vi "Main_N5224Bv5_beta.vi"() -> ()   [LabVIEW 2020]
uses:
  <instrlib>/Agilent PNA Series/Agilent PNA Series.lvlib
  Chamber_2018/ControlCluster.ctl
panel:
  out "Numeric 2":dbl
  out "Numeric":dbl
  in  "Tab Control":enum32{"Setup", "Results"}(tab)
  in  "File Path:":path=path "C:/Users/LAB543-Chamber/Desktop/meas/TEST.txt"
  in  "Saved by":string
  in  "File Description:":string
  out "error":errorcluster={"status"=FALSE, "code"=1073676294, "source"="VISA Read in MotorBack 2(SubVI).vi->Main_E8361C_2.vi"}
  in  "Cluster":T1={"Power Level"=-5.0, "Center Freq"=28000000000.0, "Span Freq"=2000000000.0, "Sweep Points"=5, "IF Bandwidth"=500.0, "Average Count"=5, "error"={"status"=FALSE, "code"=0, "source"=""}, "Instrument"="USB0::0x2A8D::0x2A01::MY58422353::INSTR", "Mode"=0, "Motor Range"=360, "Motor Step"=10, "VISA"="COM4"} {"Motor Step" items=["0.5 deg"=1, "1 deg"=2, "3 deg"=6, "5 deg"=10, "10 deg"=20]; "Motor Range" items=["360 deg"=360, "180 deg"=180]; "Mode" items=["Create", "Delete", "Select"]; "IF Bandwidth" format="%.3p"; "Span Freq" format="%.3p"; "Center Freq" format="%.3p"; "Power Level" format="%.2p"}
  out "Progress Bar":dbl(slide)=0.0055248618784530384 scale=0.0..1.0
  out "Gain array":dbl[][](array[numeric]) format="%#.3p"
  out "Gain Patten":dbl[][](graph)
  out "Phase array":dbl[][](array[numeric]) format="%#.3p"
  out "CurrentGain":dbl[](array[numeric])
  out "CurrentPhase":dbl[](array[numeric])
  # "Hz"
  # "Hz"
  # "Hz"
  # "dBm"
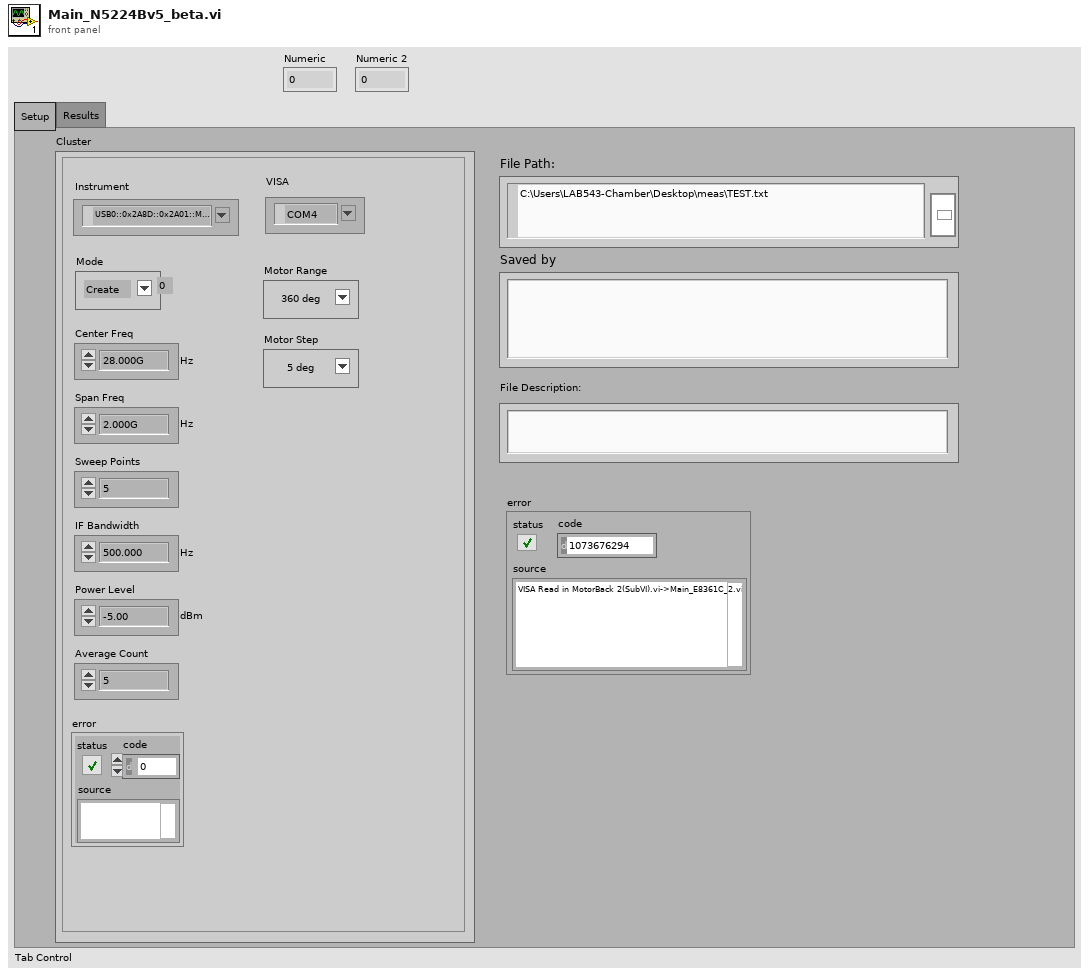
[diagram p1: front panel]
types:
  T1 = typedef "ControlCluster.ctl" = cluster{"Power Level":dbl, "Center Freq":dbl, "Span Freq":dbl, "Sweep Points":u32, "IF Bandwidth":dbl, "Average Count":i32, "error":errorcluster, "Instrument":refnum<visa-resource-name>, "Mode":u16, "Motor Range":u16, "Motor Step":u16, "VISA":refnum<visa-resource-name>}
  T2 = typedef "visaerror.ctl" = errorcluster
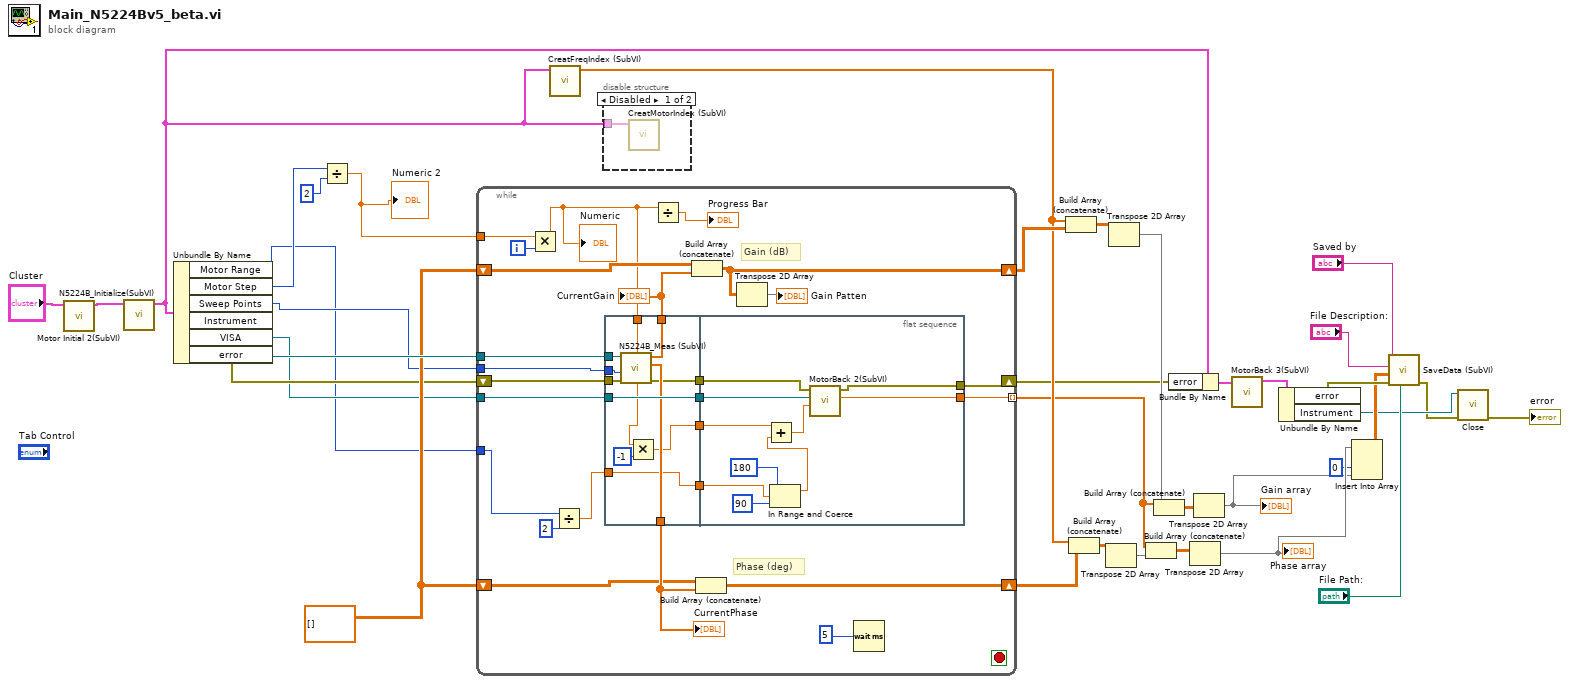
[diagram p0: block diagram]
diagram:
  w35 = dbl[][] []
  n1 = call "Motor Initial 2(SubVI).vi"("Cluster in 2"="Cluster") -> ("Cluster in 3"=w9:T1)  [unwired: 10 in]
  n2 = call "N5224B_Initialize(SubVI).vi"("Cluster in"=w9) -> ("Cluster out"=w16:T1)  [unwired: 10 in]
  n3 = Unbundle By Name(w16) -> ("Motor Range"=w2:u16, "Motor Step"=w8:u16, "Sweep Points"=w10:u32, "Instrument"=w36:refnum<visa-resource-name>, "VISA"=w6:refnum<visa-resource-name>, "error"=w7:errorcluster)
  n4 = Divide(x=w8, y=u16 2) -> (x/y=w3:dbl)
  "Numeric 2" <- w3
  n5 = while {
    tunnel: w36 -> [w61]
    shift-right: [w53] -> w33
    shift-left: w35 -> [w59]
    shift-right: [w57] -> w31
    shift-left: w35 -> [w56]
    shift-right: [w45] -> w5
    shift-left: w7 -> [w60]
    tunnel: w6 -> [w51]
    tunnel: w10 -> [w46]
    tunnel: w3 -> [w43]
    tunnel: w2 -> [w38]
    tunnel: [w37] -> w1 mode=indexing
    i -> [w49]
    stop <- _ stop-if-true
    # "Gain (dB)"
    # "Phase (deg)"
    n6 = Multiply(x=w43, y=w49) -> (x*y=w42:dbl)
    "Numeric" <- w42
    n7 = Divide(x=w38, y=2) -> (x/y=w40:dbl)
    n8 = flat-sequence {
      tunnel: w61 -> [w71]
      tunnel: w60 -> [w70]
      tunnel: [w69] -> w54
      tunnel: [w68] -> w58
      tunnel: [w67] -> w55
      tunnel: w51 -> [w72]
      tunnel: [w72] -> w50
      tunnel: w46 -> [w66]
      tunnel: [w63] -> w44
      tunnel: w42 -> [w64]
      tunnel: [w65] -> w41
      tunnel: w40 -> [w65]
      tunnel: w55 -> [w82]
      tunnel: w50 -> [w80]
      tunnel: [w81] -> w45
      tunnel: w44 -> [w75]
      tunnel: w41 -> [w77]
      tunnel: [w73] -> w37
      frame #0 {
        n9 = call "N5224B_Meas (SubVI).vi"("error in (no error)"=w70, "Sample Count (401)"=w66, "VISA Refnum in"=w71) -> ("Error Out"=w67:errorcluster, "Phase"=w68:dbl[], "Gain"=w69:dbl[])  [unwired: 6 in]
        n10 = Multiply(x=w64, y=-1) -> (x*y=w63:dbl)
      }
      frame #1 {
        n11 = In Range and Coerce(upper limit=180, x=w77, lower limit=90) -> (coerced(x)=w76:dbl)  [unwired: 1 out]
        n12 = Add(x=w75, y=w76) -> (x+y=w74:dbl)
        n13 = call "MotorBack 2(SubVI).vi"("y"=w74, "COM"=w80, "error"=w82) -> ("Locat"=w73:dbl, "error 2"=w81:T2)  [unwired: 7 in]
      }
    }
    n14 = Divide(x=w42) -> (x/y=→"Progress Bar":dbl)  [unwired: 1 in]
    n15 = Build Array (concatenate)(w59, w54) -> (w53:dbl[][])
    n16 = Build Array (concatenate)(w56, w58) -> (w57:dbl[][])
    n17 = Transpose 2D Array(2D array=w53) -> (transposed array=→"Gain Patten":dbl[][])
    n18 = Wait (ms)(milliseconds to wait=u32 5) -> ()  [unwired: 1 out]
    "CurrentGain" <- w54
    "CurrentPhase" <- w58
  }
  n19 = call "CreatFreqIndex (SubVI).vi"("Cluster in"=w16) -> ("FreqIndex"=w29:dbl[])  [unwired: 10 in]
  n20 = disable-structure shown="Disabled" {
    disable-tunnel: w16 -> [w83 _]
    frame Disabled {
      n21 = call "CreatMotorIndex (SubVI).vi"("Cluster in"=w83) -> ()  [unwired: 10 in, 1 out]
    }
    frame Enabled {
    }
  }
  n22 = Build Array (concatenate)(w29, w33) -> (w34:dbl[][])
  n23 = Build Array (concatenate)(w29, w31) -> (w32:dbl[][])
  n24 = Transpose 2D Array(2D array=w32) -> (transposed array=w30:dbl[][])
  n25 = Transpose 2D Array(2D array=w34) -> (transposed array=w28:dbl[][])
  n26 = Build Array (concatenate)(w1, w30) -> (w22:dbl[][])
  n27 = Build Array (concatenate)(w1, w28) -> (w21:dbl[][])
  n28 = Bundle By Name(cluster=w16, "error"=w5) -> (w4:T1)
  n29 = Transpose 2D Array(2D array=w22) -> (transposed array=w20:dbl[][])
  "Phase array" <- w20
  n30 = Transpose 2D Array(2D array=w21) -> (transposed array=w19:dbl[][])
  "Gain array" <- w19
  n31 = call "MotorBack 3(SubVI).vi"("Cluster in 2"=w4) -> ("Cluster in 3"=w23:T1)  [unwired: 10 in]
  n32 = Unbundle By Name(w23) -> ("error"=w27:errorcluster, "Instrument"=w15:refnum<visa-resource-name>)
  n33 = Insert Into Array(array=w20, index (col)=0 ("disabled index (col)"), new element=w19) -> (w18:dbl[][])  [unwired: 1 in]
  n34 = call "SaveData (SubVI).vi"("File Path:"="File Path:", "error in (no error)"=w27, "Data"=w18, "File \nDescription:"="File Description:", "Saved by"="Saved by") -> ("error out"=w14:errorcluster)  [unwired: 6 in]
  n35 = call <instrlib>:"Close.vi"("Error In (no error)"=w14, "VISA Resource Name"=w15) -> ("Error Out"=→"error":errorcluster)  [unwired: 9 in]
